vi "cavity_model.vi"(0 "Ir":fxp<+/-,16,14>, 2 "Ii":fxp<+/-,16,14>, 5 "input valid":bool=TRUE, 6 "reset":bool=TRUE, 7 "C3":fxp<+/-,32,3>=-2.180195599794388 format="%#_30g", 8 "C1":fxp<+/-,32,1>=0.9986428320407867, 9 "C4":fxp<+/-,32,1>=0.999985234811902, 10 "C2":fxp<+/-,32,3>=0.002117181196808815 format="%#_30g", 11 "C5":fxp<+/-,32,-32>=-5.4794710435679406e-14 format="%#_60g") -> (14 "Vr":fxp<+/-,16,14>, 16 "Vi":fxp<+/-,16,14>, 19 "output valid":bool)   [LabVIEW 2013]
uses:
  <vilib>/rvi/FXPMathLib/FxpConvert/subVIs/nifxpmath_Convert_SimConfig.ctl
  <vilib>/fxp/LVFixedPointQuantizationPolicyTypeDef.ctl
  <vilib>/fxp/LVFixedPointOverflowPolicyTypeDef.ctl
  <vilib>/rvi/FXPMathLib/FxpConvert/simVIs/DllFxpConvertTemp_sub.vi
  <vilib>/rvi/FXPMathLib/FxpConvert/XNode/nifxpmath_Convert.xnode
  <vilib>/rvi/FXPMathLib/FxpMul/XNode/nifxpmath_Multiplier.xnode
  <vilib>/rvi/FXPMathLib/FxpAdd/XNode/nifxpmath_Add.xnode
  <vilib>/rvi/FXPMathLib/sim/FxpSim.dll
panel:
  # "1-w12*dt = 0.998643"
  # "Rl*w12*dt*(10^-9) = 0.0021171821211066989"
  # "-ww1*dt = -2.1801956"
  # "1-(w1/Q1)*dt = 0.999985234514528140"
  # "C5 = (-wwK1*dt*dt/10.0.^12)*1e6 =-5.47943E-14"
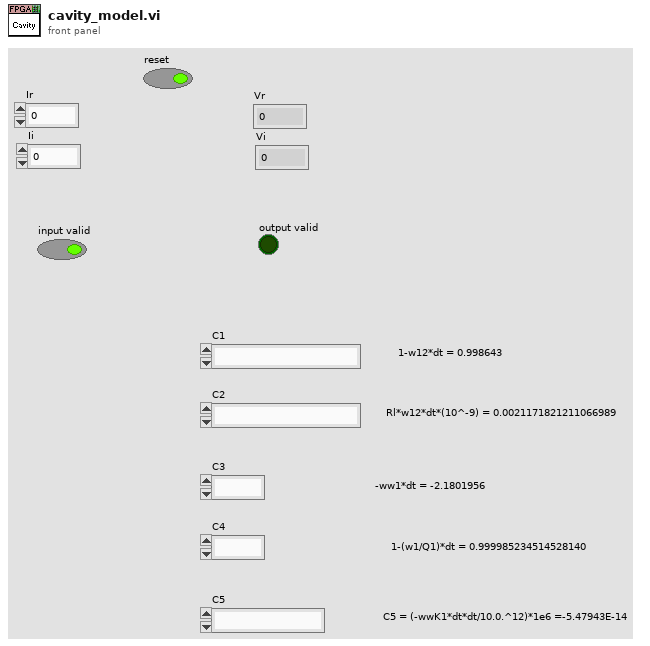
[diagram p1: front panel]
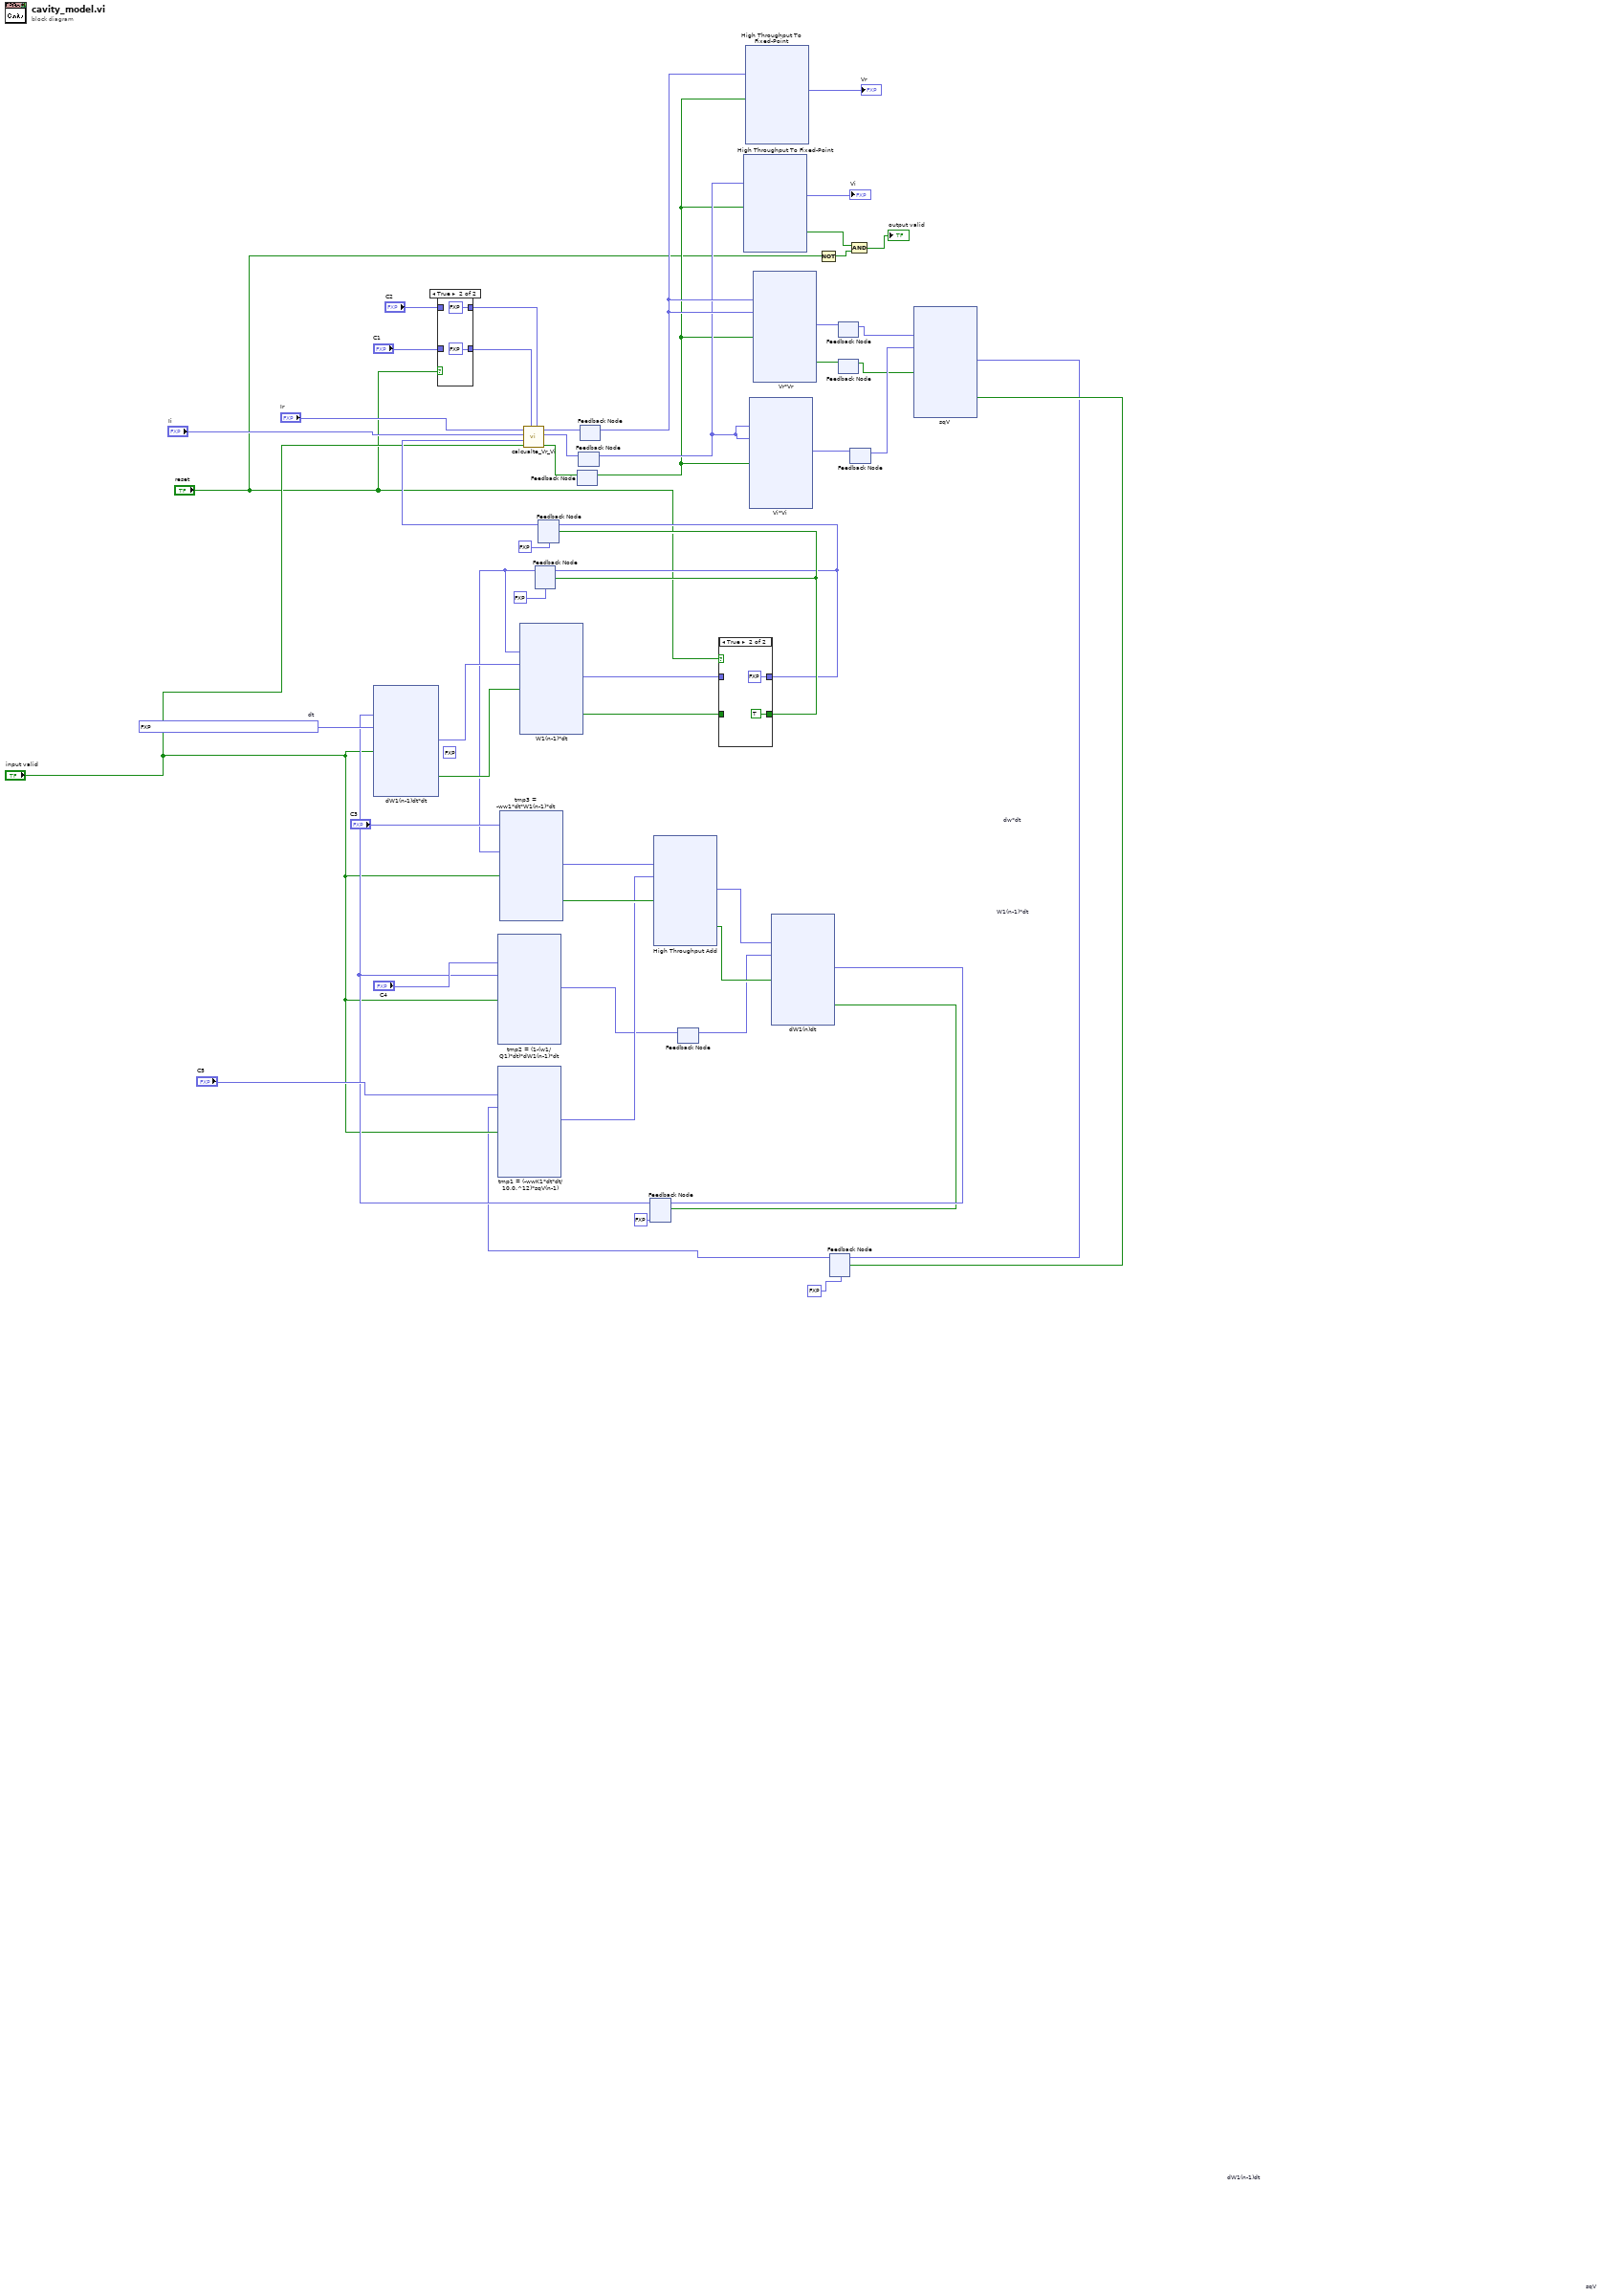
[diagram p0: block diagram]
diagram:
  (unwired) fxp<+/-,32,-12> 0.0 ("x*y")
  w53 = fxp<+/-,32,-16> 1.0000000116860974e-07  # dt
  n1 = case shown="True" "reset" {
    tunnel: "C2" -> [w56 _]
    tunnel: "C1" -> [w55 _]
    tunnel: [w56 fxp<+/-,32,3> 0.0 ("C2")] -> w6
    tunnel: [w55 fxp<+/-,32,1> 0.0 ("C1")] -> w5
    frame False {
    }
    frame True {
    }
  }
  n2 = feedback #1 "W1(n-1)*dt"(fxp<+/-,48,0> 0.0 ("dt")) -> (w46:fxp<+/-,48,0>)
  n3 = xnode "tmp3 = -ww1*dt*W1(n-1)*dt"("x"="C3", "y"=w46, "input valid"="input valid") -> ("x*y"=w31:fxp<+/-,48,-4>, "output valid"=w45:bool)  [unwired: 1 in, 1 out]
  n4 = feedback #2 "dw*dt"(fxp<+/-,48,0> 0.0 ("x")) -> (w40:fxp<+/-,48,0>)
  n5 = call "calcualte_Vr_Vi.vi"("C2"=w6, "C1"=w5, "input valid"="input valid", "dw*dt"=w40, "Ii"="Ii", "Ir"="Ir") -> ("output valid"=w19:bool, "Vi"=w21:fxp<+/-,48,16>, "Vr"=w23:fxp<+/-,48,16>)  [unwired: 3 in]
  n6 = feedback #3() -> (w18:bool)  [unwired: 1 in]
  n7 = feedback-in #3(w19) -> ()
  n8 = feedback #4() -> (w20:fxp<+/-,48,16>)  [unwired: 1 in]
  n9 = feedback-in #4(w21) -> ()
  n10 = feedback #5() -> (w22:fxp<+/-,48,16>)  [unwired: 1 in]
  n11 = feedback-in #5(w23) -> ()
  n12 = feedback #6 "dW1(n-1)dt"(fxp<+/-,48,10> 0.0 ("x")) -> (w34:fxp<+/-,48,10>)
  n13 = xnode "dW1(n-1)dt*dt"("x"=w34, "y"=w53, "input valid"="input valid") -> ("x*y"=w52:fxp<+/-,48,-16>, "output valid"=w50:bool)  [unwired: 1 in, 1 out]
  n14 = xnode "tmp2 = (1-(w1/Q1)*dt)*dW1(n-1)*dt"("x"="C4", "y"=w34, "input valid"="input valid") -> ("x*y"=w26:fxp<+/-,48,10>)  [unwired: 1 in, 2 out]
  n15 = xnode "W1(n-1)*dt"("x"=w46, "y"=w52, "input valid"=w50) -> ("x+y"=w17:fxp<+/-,48,0>, "output valid"=w16:bool)  [unwired: 1 in, 1 out]
  n16 = feedback-in #7(w26) -> ()
  n17 = feedback #7() -> (w32:fxp<+/-,48,10>)  [unwired: 1 in]
  n18 = case shown="True" "reset" {
    tunnel: w17 -> [w60 _]
    tunnel: w16 -> [w59 _]
    tunnel: [w60 fxp<+/-,48,0> 0.0 ("x+y")] -> w9
    tunnel: [w59 TRUE ("output valid")] -> w10
    frame False {
    }
    frame True {
    }
  }
  n19 = feedback-in #1(w9, w10) -> ()
  n20 = feedback-in #2(w9, w10) -> ()
  n21 = xnode "High Throughput To Fixed-Point"("x"=w20, "input valid"=w18) -> ("y"=→"Vi":fxp<+/-,16,14>, "output valid"=w4:bool)  [unwired: 1 in, 1 out]
  n22 = xnode "High Throughput To Fixed-Point"("x"=w22, "input valid"=w18) -> ("y"=→"Vr":fxp<+/-,16,14>)  [unwired: 1 in, 2 out]
  n23 = xnode "Vi*Vi"("x"=w20, "y"=w20, "input valid"=w18) -> ("x*y"=w29:fxp<+,48,32>)  [unwired: 1 in, 2 out]
  n24 = xnode "Vr*Vr"("x"=w22, "y"=w22, "input valid"=w18) -> ("x*y"=w28:fxp<+/-,48,32>, "output valid"=w39:bool)  [unwired: 1 in, 1 out]
  n25 = Not(x="reset") -> (.not. x?=w2:bool)
  n26 = feedback #8 "sqV"(fxp<+/-,48,32> 0.0 ("x")) -> (w30:fxp<+/-,48,32>)
  n27 = xnode "tmp1 = (-wwK1*dt*dt/10.0.^12)*sqV(n-1)"("x"="C5", "y"=w30, "input valid"="input valid") -> ("x*y"=w27:fxp<+/-,48,-4>)  [unwired: 1 in, 2 out]
  n28 = xnode ("High Throughput Add")("x"=w31, "y"=w27, "input valid"=w45) -> ("x+y"=w35:fxp<+/-,48,-2>, "output valid"=w44:bool)  [unwired: 1 in, 1 out]
  n29 = xnode "dW1(n)dt"("x"=w35, "y"=w32, "input valid"=w44) -> ("x+y"=w15:fxp<+/-,48,10>, "output valid"=w14:bool)  [unwired: 1 in, 1 out]
  n30 = feedback-in #6(w15, w14) -> ()
  n31 = feedback #9() -> (w38:fxp<+/-,48,32>)  [unwired: 1 in]
  n32 = feedback-in #9(w28) -> ()
  n33 = feedback #10() -> (w36:bool)  [unwired: 1 in]
  n34 = feedback-in #10(w39) -> ()
  n35 = And(x=w4, y=w2) -> (x .and. y?=→"output valid":bool)
  n36 = feedback #11() -> (w37:fxp<+,48,32>)  [unwired: 1 in]
  n37 = feedback-in #11(w29) -> ()
  n38 = xnode "sqV"("x"=w38, "y"=w37, "input valid"=w36) -> ("x+y"=w11:fxp<+/-,48,32>, "output valid"=w13:bool)  [unwired: 1 in, 1 out]
  n39 = feedback-in #8(w11, w13) -> ()
